vi "Handle Error.vi"(8 "error in (no error)":errorcluster, 11 "Root Panel Actor in":refnum<class "Root Panel Actor.lvclass">) -> (0 "error out":errorcluster, 2 "stop actor?":bool=TRUE, 3 "Root Panel Actor out":refnum<class "Root Panel Actor.lvclass">)   [LabVIEW 2021, in "Root Panel.lvlib" / "Root Panel Actor.lvclass"]
doc: "(<B>Filename</B>: Actor Framework.lvlib:Actor.lvclass:Handle Error.vi)\n\nDefines how the actor handles an error that occurred while processing a message. By default, this method does nothing except stop the actor."
uses:
  Root Panel Actor.lvclass
  Appearance Actor/Appearance Actor/Appearance Actor.lvclass
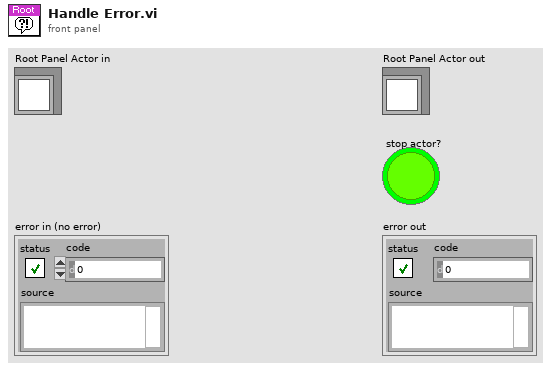
[diagram p1: front panel]
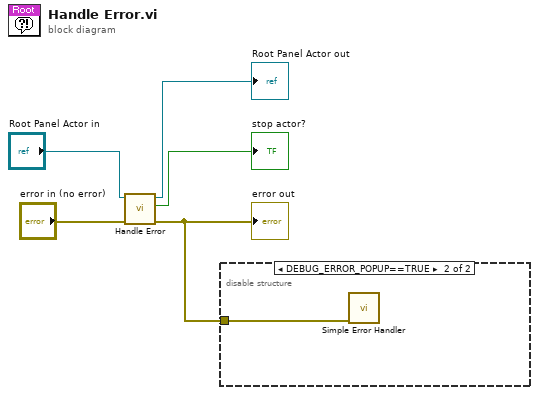
[diagram p0: block diagram]
diagram:
  n1 = call-parent "Handle Error.vi"("error in (no error)"="error in (no error)", "Actor in"="Root Panel Actor in") -> ("error out"=w2:errorcluster, "stop actor?"=→"stop actor?":bool, "Actor out"=→"Root Panel Actor out":refnum<class "Root Panel Actor.lvclass">)  [unwired: 7 in]
  "error out" <- w2
  n2 = disable-structure shown="DEBUG_ERROR_POPUP==TRUE" {
    disable-tunnel: w2 -> [_ w6]
    frame condition #0 {
    }
    frame condition #1 (active) {
      n3 = call <vilib>:"Simple Error Handler.vi"("error in (no error)"=w6) -> ()  [unwired: 4 in, 5 out]
    }
  }
